vi "Word to Float.vi"(1 "Range":sgl=1.0, 2 "Word (string, big endian)":string="\u0000\u0000") -> (0 "float32 out":sgl)   [LabVIEW 2015]
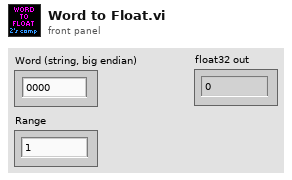
[diagram p1: front panel]
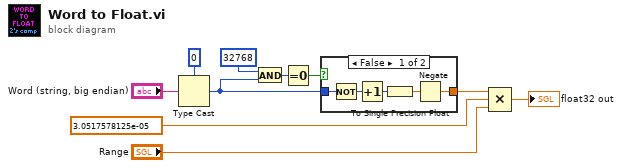
[diagram p0: block diagram]
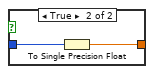
[diagram p2: hidden frame]
diagram:
  n1 = Type Cast(type=u16 0, x="Word (string, big endian)") -> (*(type *) &x=w1:u16)
  n2 = And(x=u16 32768, y=w1) -> (x .and. y?=w3:u16)
  n3 = Equal To 0?(x=w3) -> (x = 0?=w2:bool)
  n4 = case shown="False" w2 {
    tunnel: [w13 w16] -> w5
    tunnel: w1 -> [w12 w17]
    frame False {
      n5 = Not(x=w12) -> (.not. x?=w11:u16)
      n6 = Increment(x=w11) -> (x+1=w14:u16)
      n7 = To Single Precision Float(number=w14) -> (single precision float=w15:sgl)
      n8 = Negate(x=w15) -> (-x=w13:sgl)
    }
    frame True {
      n9 = To Single Precision Float(number=w17) -> (single precision float=w16:sgl)
    }
  }
  n10 = Compound Arithmetic op=MULTIPLY(w5, sgl 3.0517578e-05 ("1/x"), "Range") -> (→"float32 out":sgl)
